vi "RT_Control_AllIncluded_AngleToPy.vi"(10 "rt fifo":refnum<k33>, 11 "Parameters":T1) -> (0 "error out":errorcluster, 2 "Delayed Cycles":dbl)   [LabVIEW 2021]
uses:
  parametersRT.ctl
  <vilib>/DAQmx/write.llb/DAQmx Write (Analog 1D DBL NChan 1Samp).vi
  <vilib>/DAQmx/read.llb/DAQmx Read (Analog 1D DBL NChan 1Samp).vi
  <vilib>/DAQmx/configure/timing.llb/DAQmx Timing (Sample Clock).vi
  <vilib>/DAQmx/miscellaneous.llb/DAQmx Fill In Error Info.vi
  <resource>/objmgr/daqmx.rc
panel:
  out "size(s)":i32
  out "ESP array size":i32
  out "error out 7":errorcluster
  out "error out 6":errorcluster
  out "error out 5":errorcluster
  out "error out 4":errorcluster
  out "error out 3":errorcluster
  out "error out 2":errorcluster
  out "FB Raw Readings":dbl[][](array[numeric])
  in  "System Information":enum32{"RT System"}(tab)
  in  "source":tag
  in  "source 2":tag
  in  "Stop Loop":bool
  in  "RT Data Monitoring":enum32{"Forces", "Angles", "Power", "Pressure"}(tab)
  out "Bias Voltages":dbl[][](array[numeric])=[[-0.0710179470114859, -0.17463349299050945, -0.11016159714741332, 0.026018829634351103, 0.12897648926553976, 0.08259620236774425]]
  out "Bias Vector":dbl[](array[numeric])=[-0.0710179470114859, -0.17463349299050945, -0.11016159714741332, 0.026018829634351103, 0.12897648926553976, 0.08259620236774425]
  in  "Bias":bool
  in  "Unbias":bool
  out "ESP 2":sgl[][](array[numeric])
  # "Important! Set angle offset before reading angles"
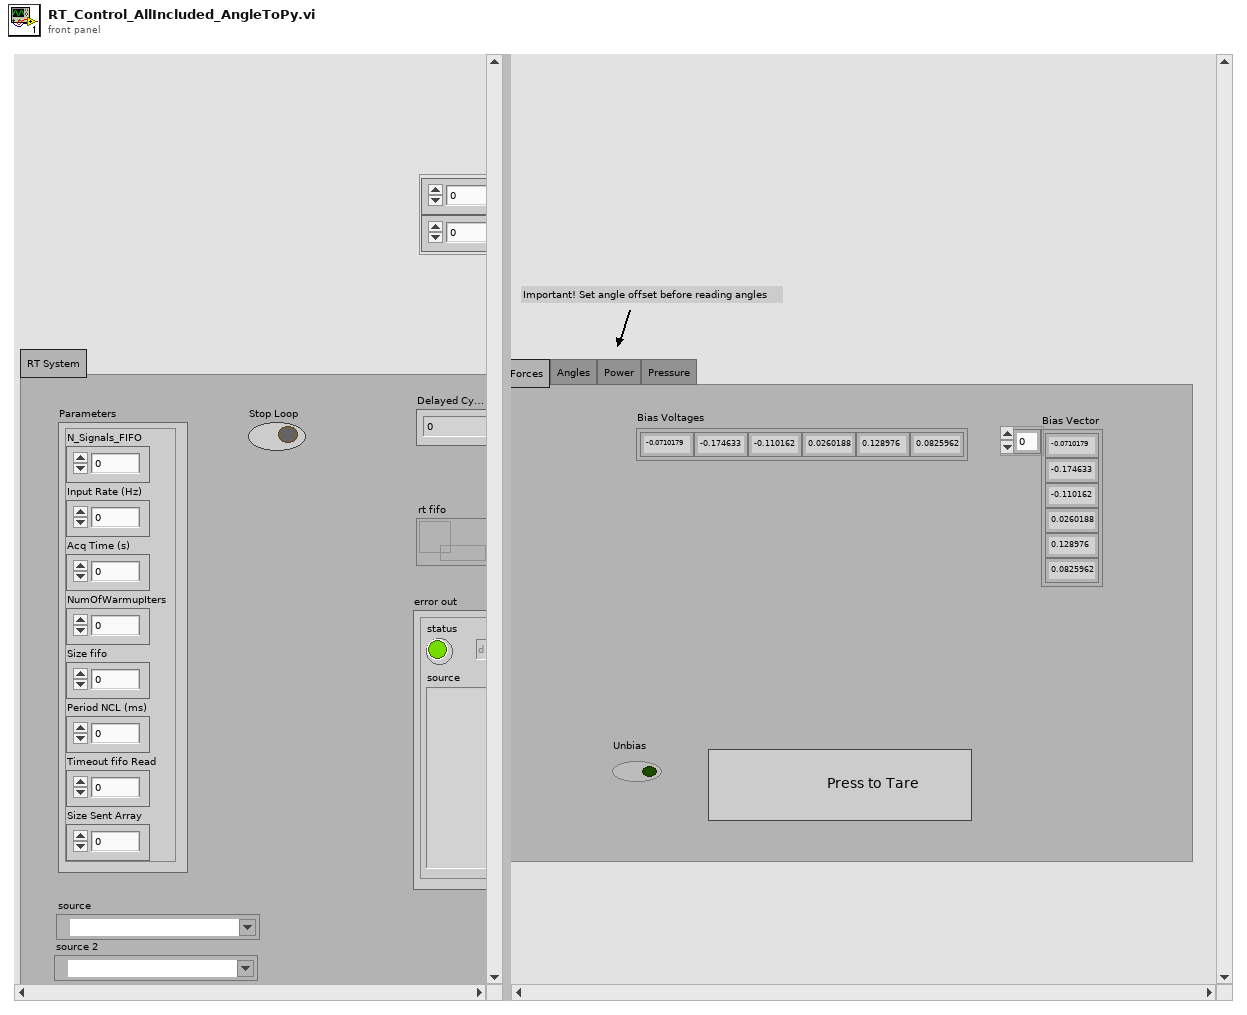
[diagram p1: front panel]
types:
  T1 = typedef "parametersRT.ctl" = cluster{"N_Signals_FIFO":u32, "Input Rate (Hz)":dbl, "Acq Time (s)":dbl, "NumOfWarmupIters":u32, "Size fifo":u32, "Period NCL (ms)":i64, "Timeout fifo Read":i32, "Size Sent Array":i32}
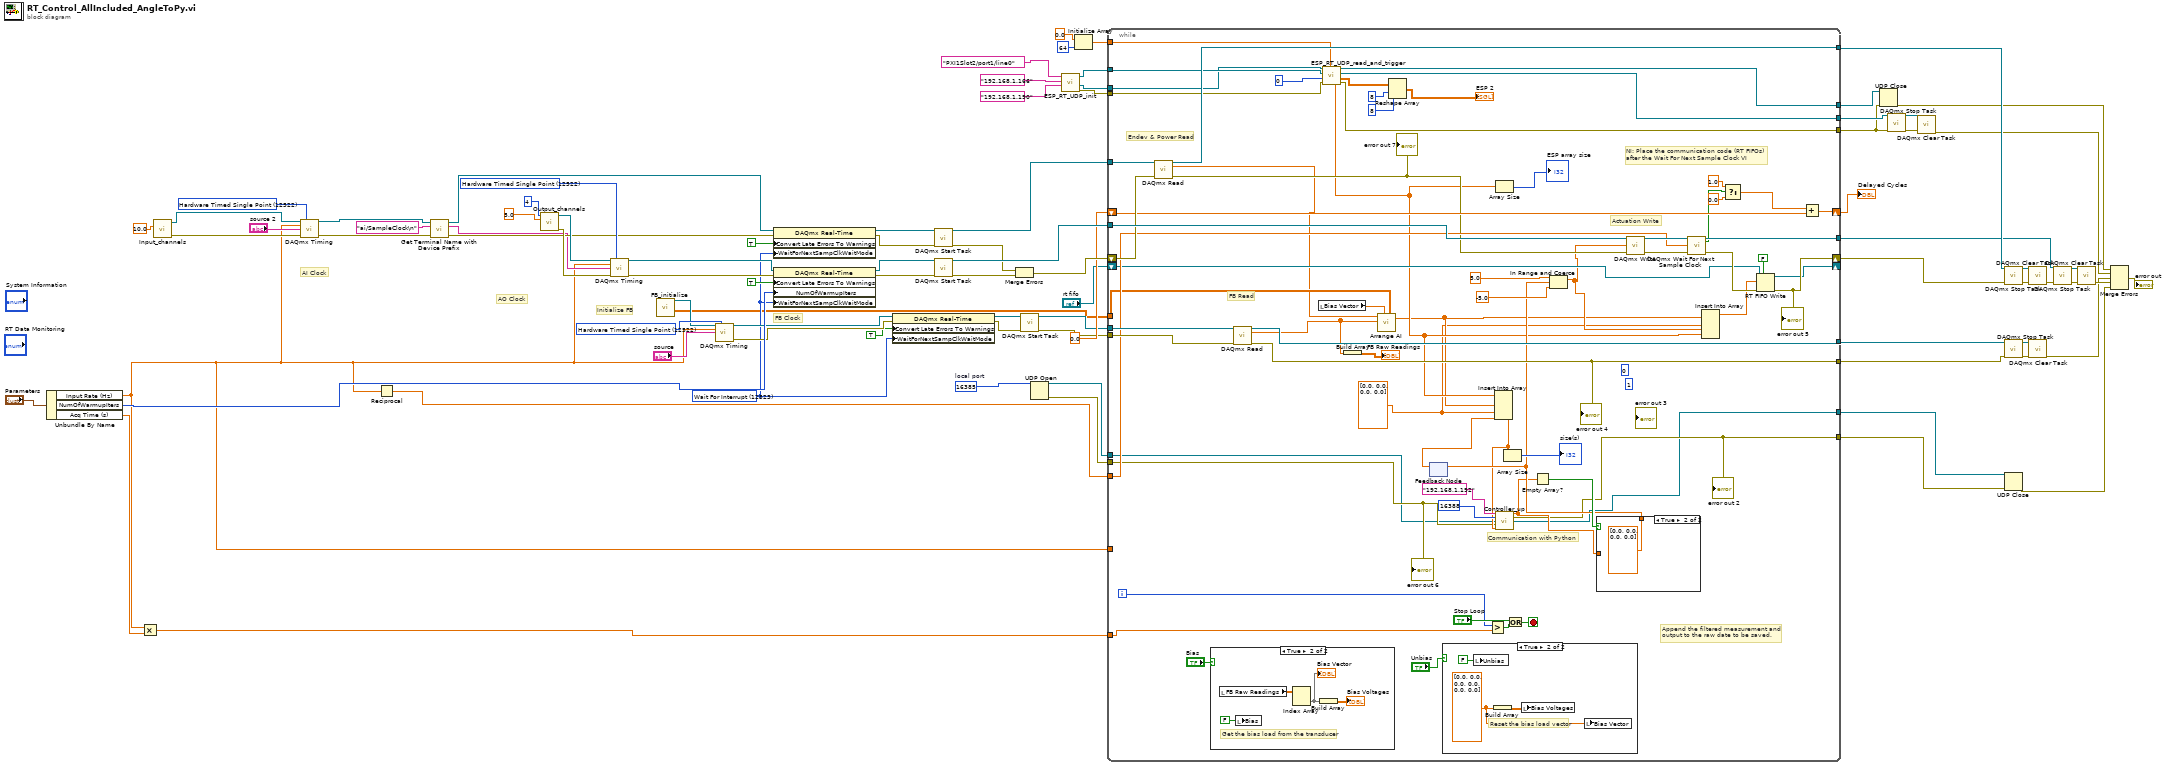
[diagram p0: block diagram]
diagram:
  w50 = 12522 items=["Finite Samples"=10178, "Continuous Samples"=10123, "Hardware Timed Single Point"=12522] ("sample mode")
  w60 = u16 16385  # local port
  w67 = 12522 items=["Finite Samples"=10178, "Continuous Samples"=10123, "Hardware Timed Single Point"=12522] ("sample mode")
  w45 = 12523 items=["Wait For Interrupt"=12523, "Poll"=12524, "Yield"=12525] ("WaitForNextSampClkWaitMode")
  w86 = 12522 items=["Finite Samples"=10178, "Continuous Samples"=10123, "Hardware Timed Single Point"=12522] ("sample mode")
  # "Initialize FB"
  # "AO Clock"
  # "AI Clock"
  # "FB Clock"
  n1 = Unbundle By Name("Parameters") -> ("Input Rate (Hz)"=w18:dbl, "NumOfWarmupIters"=w74:u32, "Acq Time (s)"=w80:dbl)
  n2 = Multiply(x=w18, y=w80) -> (x*y=w55:dbl)
  n3 = call "Input_channels.vi"("Range"=10.0) -> ("error out"=w69:errorcluster, "Refnum out"=w68:refnum<k21>)  [unwired: 9 in]
  n4 = call-poly <vilib>:"DAQmx Timing.vi"("task/channels in"=w68, "sample mode"=w67, "rate"=w18, "source"="source 2", "error in"=w69) -> ("task out"=w38:refnum<k21>, "error out"=w36:errorcluster)  [unwired: 9 in]
  n5 = Reciprocal(x=w18) -> (1/x=w85:dbl)
  n6 = call "Get Terminal Name with Device Prefix.vi"("error in (no error)"=w36, "Local Terminal Name"="ai/SampleClock\n", "task/channels in"=w38) -> ("error out"=w35:errorcluster, "Terminal Name with Device Prefix"=w34:tag, "task out"=w37:refnum<k21>)  [unwired: 6 in]
  n7 = call "Output_channels.vi"(10:5.0 ("Maximum Value"), "nchan"=4) -> ("error out"=w77:errorcluster, "Refnum out"=w76:refnum<k21>)  [unwired: 8 in]
  n8 = call-poly <vilib>:"DAQmx Timing.vi"("task/channels in"=w76, "sample mode"=w86, "rate"=w18, "source"=w34, "error in"=w77) -> ("task out"=w84:refnum<k21>, "error out"=w83:errorcluster)  [unwired: 9 in]
  n9 = call "FB_initialize.vi"() -> ("Transformed Calibration Matrix"=w42:dbl[][], "FB out"=w46:refnum<k21>)  [unwired: 9 in, 1 out]
  n10 = call-poly <vilib>:"DAQmx Timing.vi"("task/channels in"=w46, "sample mode"=w50, "rate"=w18, "source"="source") -> ("task out"=w52:refnum<k21>, "error out"=w51:errorcluster)  [unwired: 10 in]
  n11 = property class="DAQmx Real-Time"(reference=w37, error in=w35, "Convert Late Errors To Warnings"=TRUE, "WaitForNextSampClkWaitMode"=w45) -> (reference out=w64:refnum<k21>, error out=w63:errorcluster)
  n12 = property class="DAQmx Real-Time"(reference=w84, error in=w83, "Convert Late Errors To Warnings"=TRUE, "NumOfWarmupIters"=w74, "WaitForNextSampClkWaitMode"=w45) -> (reference out=w81:refnum<k21>, error out=w71:errorcluster)
  n13 = property class="DAQmx Real-Time"(reference=w52, error in=w51, "Convert Late Errors To Warnings"=TRUE ("ConvLateErrorsToWarnings"), "WaitForNextSampClkWaitMode"=w45) -> (reference out=w47:refnum<k21>, error out=w48:errorcluster)
  n14 = call <vilib>:"DAQmx Start Task.vi"("task/channels in"=w64, "error in"=w63) -> ("task out"=w79:refnum<k21>, "error out"=w62:errorcluster)  [unwired: 12 in]
  n15 = call <vilib>:"DAQmx Start Task.vi"("task/channels in"=w81, "error in"=w71) -> ("task out"=w78:refnum<k21>, "error out"=w70:errorcluster)  [unwired: 12 in]
  n16 = Merge Errors(w62, w70) -> (w61:errorcluster)
  n17 = call <vilib>:"DAQmx Start Task.vi"("task/channels in"=w47, "error in"=w48) -> ("task out"=w44:refnum<k21>, "error out"=w43:errorcluster)  [unwired: 12 in]
  n18 = UDP Open(11:w60) -> (port=w58:refnum<k16>, 0:w59:errorcluster)  [unwired: 4 in, 1 out]
  n19 = call "ESP_RT_UDP_init.vi"("Trigger Port"=tag "PXI1Slot2/port1/line0" ("lines"), "PXI(local) IP"="192.168.1.166" ("Hardware Trigger"), "ESP(remote) IP"="192.168.1.190" ("IP address")) -> ("task out"=w12:refnum<k21>, "connection ID out"=w11:refnum<k16>, "error out"=w13:errorcluster)  [unwired: 5 in]
  n20 = Initialize Array(0.0, 64) -> (w8:dbl[])
  n21 = while {
    shift-right: [w133] -> w27
    shift-left: w61 -> [w147]
    shift-right: [w152] -> w87
    shift-left: 0.0 ("f") -> [w146]
    tunnel: w85 -> [w135]
    tunnel: w55 -> [w151]
    tunnel: w78 -> [w150]
    tunnel: [w148] -> w26
    tunnel: w79 -> [w149]
    tunnel: [w137] -> w22
    tunnel: w59 -> [w89]
    tunnel: w58 -> [w88]
    tunnel: [w90] -> w57
    tunnel: w44 -> [w145]
    tunnel: w43 -> [w144]
    tunnel: w42 -> [w123]
    tunnel: [w141] -> w32
    tunnel: [w140] -> w30
    shift-right: [w131] -> _
    shift-left: "rt fifo" -> [w130]
    tunnel: [w91] -> w19
    tunnel: w18 -> [_]
    tunnel: w13 -> [w115]
    tunnel: w12 -> [w114]
    tunnel: w11 -> [w113]
    tunnel: w8 -> [w112]
    tunnel: [w111] -> w5
    tunnel: [w110] -> w4
    tunnel: [w109] -> w3
    i -> [w118]
    stop <- w125 stop-if-true
    w96 = dbl[] [0.0, 0.0, 0.0, 0.0]
    (unwired) 1 ("length")
    (unwired) 0 ("index")
    # "NI: Place the communication code (RT FIFOs) \nafter the Wait For Next Sample Clock VI"
    # "Communication with Python"
    # "Actuation Write"
    # "Endev & Power Read"
    # "FB Read"
    # "Append the filtered measurement and \noutput to the raw date to be saved."
    n22 = call-poly <vilib>:"DAQmx Read.vi"("task/channels in"=w149, "error in"=w147) -> ("task out"=w148:refnum<k21>, "data"=w117:dbl[], "error out"=w128:errorcluster)  [unwired: 11 in]
    "error out 7" <- w128
    n23 = case shown="True" "Bias" {
      frame False {
      }
      frame True {
        # "Get the bias load from the transducer"
        n24 = local read "FB Raw Readings"() -> (w164:dbl[][])
        n25 = local write "Bias"(FALSE) -> ()
        n26 = Index Array(array=w164) -> (element=w161:dbl[])  [unwired: 2 in]
        "Bias Vector" <- w161
        n27 = Build Array(w161) -> (→"Bias Voltages":dbl[][])
      }
    }
    n28 = call-poly <vilib>:"DAQmx Read.vi"("task/channels in"=w145, "error in"=w144) -> ("task out"=w141:refnum<k21>, "data"=w122:dbl[], "error out"=w140:errorcluster)  [unwired: 11 in]
    "error out 4" <- w140
    n29 = local read "Bias Vector"() -> (w124:dbl[])
    n30 = call "ESP_RT_UDP_read_and_trigger.vi"("Data_In"=w112, "error in"=w115, "UDP_read_timeout(ms)"=0, "Trigger_task_in"=w114, "connection ID"=w113) -> ("error out"=w109:errorcluster, "ESP_Data(1x64)"=w100:dbl[][], "Trigger_task_out"=w110:refnum<k21>, "connection ID out"=w111:refnum<k16>, "ESP_Index_Data"=w102:dbl[])  [unwired: 1 in, 1 out]
    n31 = Build Array(w122) -> (→"FB Raw Readings":dbl[][])
    n32 = call "Arrange AI.vi"("Transformed Calibration Matrix"=w123, "Bias Vector"=w124, "FB data"=w122, "EDV + Voltage data"=w117) -> ("FIFO Data (7EDV+3Force+4Power+4Voltage)"=w101:dbl[])  [unwired: 6 in, 1 out]
    n33 = Reshape Array(w100, 8 ("dimension size"), 8 ("dimension size")) -> (→"ESP 2":dbl[][])
    n34 = feedback #1() -> (w106:dbl[])  [unwired: 1 in]
    n35 = case shown="True" "Unbias" {
      frame False {
      }
      frame True {
        w159 = dbl[] [0.0, 0.0, 0.0, 0.0, 0.0, 0.0]
        # "Reset the bias load vector"
        n36 = local write "Unbias"(FALSE) -> ()
        n37 = Build Array(w159) -> (w158:dbl[][])
        n38 = local write "Bias Voltages"(w158) -> ()
        n39 = local write "Bias Vector"(w159) -> ()
      }
    }
    n40 = Greater?(x=w118, y=w151) -> (0:w126:bool)
    n41 = Insert Into Array(array=w102, new element #1=w101, new element #2=w96, new element #3=w106) -> (w93:dbl[])  [unwired: 1 in]
    n42 = Array Size(array=w102) -> (size(s)=→"ESP array size":i32)
    n43 = call "Controller_up.vi"("name 2"="192.168.1.192", "port or service name"=u16 16388, "connection ID"=w88, "error in (no error)"=w89, "x"=w93) -> ("*(type *) &x"=w92:dbl[], "error out"=w91:errorcluster, "connection ID out"=w90:refnum<k16>)  [unwired: 8 in]
    "error out 2" <- w91
    n44 = Array Size(array=w93) -> (size(s)=→"size(s)":i32)
    n45 = Or(x="Stop Loop", y=w126) -> (x .or. y?=w125:bool)
    n46 = Empty Array?(array=w92) -> (empty?=w104:bool)
    n47 = case shown="True" w104 {
      tunnel: [w156 dbl[] [0.0, 0.0, 0.0, 0.0]] -> w103
      tunnel: w92 -> [w156 _]
      frame False {
      }
      frame True {
      }
    }
    n48 = feedback-in #1(w103) -> ()
    n49 = In Range and Coerce(upper limit=5.0, x=w103, lower limit=-5.0) -> (coerced(x)=w108:dbl[])  [unwired: 1 out]
    n50 = call-poly <vilib>:"DAQmx Write.vi"("task/channels in"=w150, "data"=w108, "error in"=w128) -> ("task out"=w138:refnum<k21>, "error out"=w139:errorcluster)  [unwired: 10 in, 1 out]
    n51 = call <vilib>:"DAQmx Wait For Next Sample Clock.vi"("task/channels in"=w138, "timeout (sec)"=w135, "error in"=w139) -> ("task out"=w137:refnum<k21>, "is late?"=w136:bool, "error out"=w132:errorcluster)  [unwired: 10 in]
    n52 = Insert Into Array(array=w101, new element #1=w96, new element #2=w108, new element #3=w102) -> (w129:dbl[])  [unwired: 1 in]
    n53 = Select(t=1.0, s=w136, f=0.0) -> (s? t:f=w153:dbl)
    n54 = RT FIFO Write(0:w130, 1:w129, 3:w132, 5:FALSE ("overwrite on timeout (T)")) -> (8:w131:refnum<k33>, 11:w133:errorcluster)  [unwired: 1 in, 2 out]
    "error out 5" <- w133
    n55 = Add(x=w153, y=w146) -> (x+y=w152:dbl)
    "error out 6" <- w89
  }
  "Delayed Cycles" <- w87
  n56 = UDP Close(connection ID=w5, 8:w3) -> (error out=w2:errorcluster)  [unwired: 1 out]
  n57 = call <vilib>:"DAQmx Stop Task.vi"("task/channels in"=w4, "error in"=w3) -> ("task out"=w6:refnum<k21>, "error out"=w7:errorcluster)  [unwired: 12 in]
  n58 = call <vilib>:"DAQmx Clear Task.vi"("task in"=w6, "error in"=w7) -> ("error out"=w1:errorcluster)  [unwired: 13 in]
  n59 = call <vilib>:"DAQmx Stop Task.vi"("task/channels in"=w26, "error in"=w27) -> ("task out"=w25:refnum<k21>, "error out"=w28:errorcluster)  [unwired: 12 in]
  n60 = call <vilib>:"DAQmx Stop Task.vi"("task/channels in"=w32, "error in"=w30) -> ("task out"=w31:refnum<k21>, "error out"=w29:errorcluster)  [unwired: 12 in]
  n61 = UDP Close(connection ID=w57, 8:w19) -> (error out=w56:errorcluster)  [unwired: 1 out]
  n62 = call <vilib>:"DAQmx Clear Task.vi"("task in"=w25, "error in"=w28) -> ("error out"=w24:errorcluster)  [unwired: 13 in]
  n63 = call <vilib>:"DAQmx Clear Task.vi"("task in"=w31, "error in"=w29) -> ("error out"=w41:errorcluster)  [unwired: 13 in]
  n64 = call <vilib>:"DAQmx Stop Task.vi"("task/channels in"=w22, "error in"=w24) -> ("task out"=w21:refnum<k21>, "error out"=w23:errorcluster)  [unwired: 12 in]
  n65 = call <vilib>:"DAQmx Clear Task.vi"("task in"=w21, "error in"=w23) -> ("error out"=w73:errorcluster)  [unwired: 13 in]
  n66 = Merge Errors(w2, w1, w41, w73, w56) -> (→"error out":errorcluster)
